vi "Close.vi"(8 "error in (no error)":errorcluster, 11 "RemoteDataService in":refnum<class "RemoteDataService.lvclass">) -> (0 "error out":errorcluster)   [LabVIEW 2020, in "Vecto.lvlib" / "RemoteDataService.lvclass"]
uses:
  RemoteDataService.lvclass
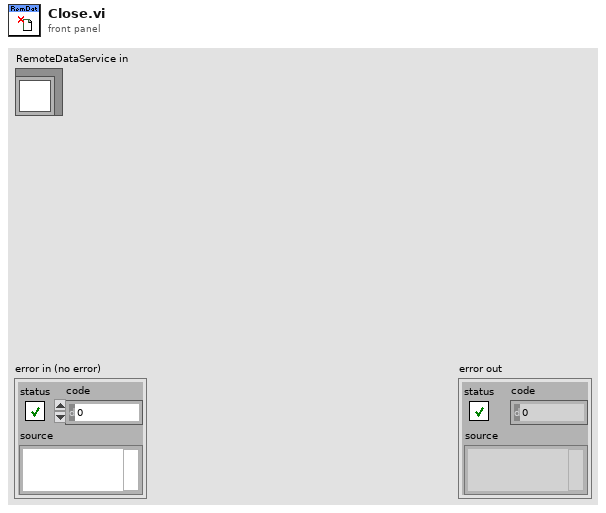
[diagram p1: front panel]
types:
  T1 = typedef "Vecto.lvlib/RemoteDataService.lvclass/Incoming Events.ctl" = cluster{"Register Group":refnum<user-event>, "Close":refnum<user-event>, "Publish Group":refnum<user-event>, "Start":refnum<user-event>, "Subscribe":refnum<user-event>, "Registered Groups":refnum<user-event>}
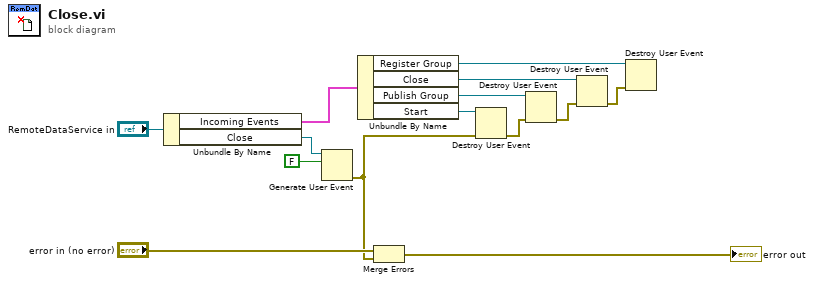
[diagram p0: block diagram]
diagram:
  n1 = Unbundle By Name("RemoteDataService in") -> ("Incoming Events"=w10:T1, "Close"=w12:refnum<user-event>)
  n2 = Generate User Event(user event=w12, event data cluster=FALSE ("event data")) -> (error out=w1:errorcluster)  [unwired: 2 in, 1 out]
  n3 = Unbundle By Name(w10) -> ("Register Group"=w4:refnum<user-event>, "Close"=w6:refnum<user-event>, "Publish Group"=w8:refnum<user-event>, "Start"=w9:refnum<user-event>)
  n4 = Merge Errors("error in (no error)", w1) -> (→"error out":errorcluster)
  n5 = Destroy User Event(user event=w9, error in=w1) -> (error out=w7:errorcluster)
  n6 = Destroy User Event(user event=w8, error in=w7) -> (error out=w5:errorcluster)
  n7 = Destroy User Event(user event=w6, error in=w5) -> (error out=w3:errorcluster)
  n8 = Destroy User Event(user event=w4, error in=w3) -> ()  [unwired: 1 out]
